vi "Digital Write Port Test.vi"() -> ()   [LabVIEW 2011]
uses:
  Private/Type Defs/Chipkit Configuration.ctl
  Private/Type Defs/Board Type.ctl
  LabVIEW Interface for ChipKit.lvlib
panel:
  in  "ChipKit Configuration":T1={"COM Port"="COM6", "Board Type"=enum."ChipKit uC32"}
  in  "Stop Button":bool
  in  "DIO Pin Values":bool[](array[boolean])=[FALSE, TRUE, FALSE]
  in  "DIO Pins":u8[](array[numeric])=[4, 5, 6]
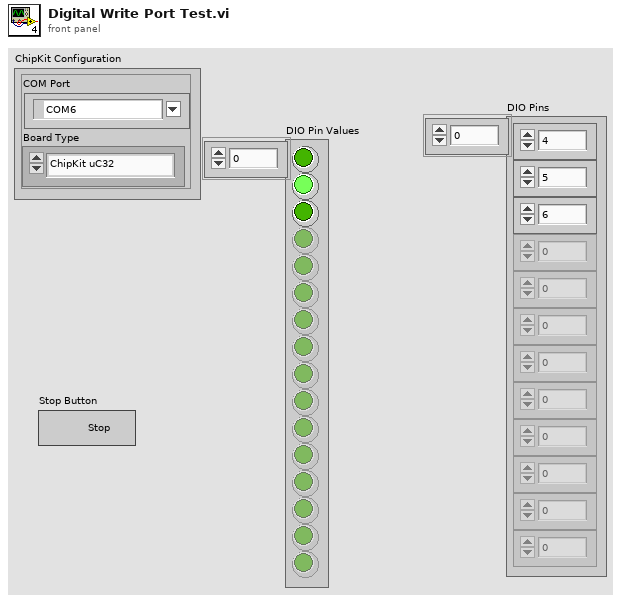
[diagram p1: front panel]
types:
  T1 = typedef "LabVIEW Interface for ChipKit.lvlib/Chipkit Configuration.ctl" = cluster{"COM Port":refnum<visa-resource-name>, "Board Type":T2}
  T2 = typedef "LabVIEW Interface for ChipKit.lvlib/Board Type.ctl" = enum16{"ChipKit uC32", "ChipKit Uno32", "ChipKit Max32"}
  T3 = typedef "LabVIEW Interface for ChipKit.lvlib/Chipkit Resource.ctl" = cluster{"COM Port":refnum<visa-resource-name>, "Board Type":T2, "Connection Type":T4, "Baud Rate (115200)":u32, "Bytes Per Packet (15)":u32, "DI Port Num Pins":i32, "DO Port Num Pins":i32}
  T4 = typedef "LabVIEW Interface for ChipKit.lvlib/Connection Type.ctl" = enum8{"USB / Serial", "XBEE", "BlueSmirf (Bluetooth)"}
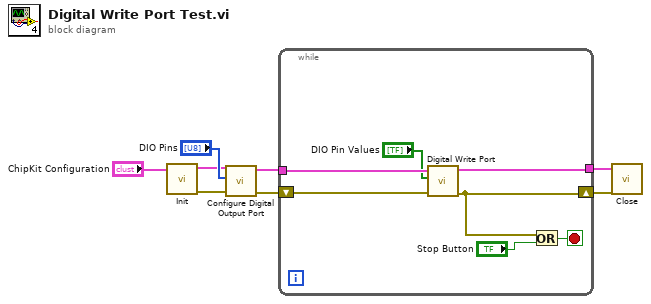
[diagram p0: block diagram]
diagram:
  n1 = call "Init.vi"("ChipKit Configuration"="ChipKit Configuration") -> ("Error Out"=w2:errorcluster, "ChipKit Configuration"=w3:T3)  [unwired: 9 in]
  n2 = call "Configure Digital Output Port.vi"("Error In"=w2, "DO Pins"="DIO Pins", "ChipKit Resource"=w3) -> ("Error Out"=w6:errorcluster, "ChipKit Resource"=w8:T3)  [unwired: 7 in]
  n3 = while {
    tunnel: w8 -> [w15]
    tunnel: [w14] -> w7
    shift-right: [w10] -> w5
    shift-left: w6 -> [w13]
    stop <- w11 stop-if-true
    n4 = call "Digital Write Port.vi"("Error In"=w13, "DO Pin Values"="DIO Pin Values", "ChipKit Resource"=w15) -> ("Error Out"=w10:errorcluster, "ChipKit Resource"=w14:T3)  [unwired: 7 in]
    n5 = Or(x=w10, y="Stop Button") -> (x .or. y?=w11:bool)
  }
  n6 = call "Close.vi"("Error In"=w5, "ChipKit Configuration"=w7) -> ()  [unwired: 9 in, 1 out]
